vi "Create Actor.vi"(11 "QualifiedName":string="demo/producer") -> (0 "error out":errorcluster, 3 "Actor Class":T1)   [LabVIEW 2013]
uses:
  Actor Private Data.ctl
  <vilib>/LabVIEW Open Source Project/MQTT Client/Client class/Client.lvclass
  Actor Private Events -- cluster.ctl
  Payload -- cluster.ctl
  <vilib>/LabVIEW Open Source Project/OpenSerializer JKI JSON/Serializer.JSON.lvclass
  <vilib>/LabVIEW Open Source Project/MQTT Connection/MQTT_Base/Base Class/MQTT_Base.lvclass/MQTT_Base.ctl
  <vilib>/LabVIEW Open Source Project/MQTT Control Packets/Control Packets/PUBLISH/PUBLISH.lvclass
  <vilib>/LabVIEW Open Source Project/OpenSerializer/Serializer.FlattenedString/Serializer.FlattenedString.lvclass
  <vilib>/LabVIEW Open Source Project/OpenSerializer/Serializer/Serializer.lvclass
  <vilib>/LabVIEW Open Source Project/Connection/Connection.TCP/Connection.TCP.lvclass
  <vilib>/LabVIEW Open Source Project/MQTT Connection/MQTT_Base/Base Class/MQTT_Base.lvclass
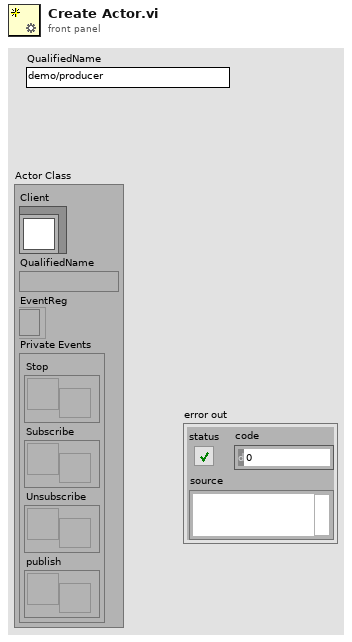
[diagram p1: front panel]
types:
  T1 = typedef "Actor Private Data.ctl" = cluster{"Client":refnum<class "Client.lvclass">, "QualifiedName":string, "EventReg":refnum<event-registration>, "Private Events":T2}
  T2 = typedef "Actor Private Events -- cluster.ctl" = cluster{"Stop":refnum<user-event>, "Subscribe":refnum<user-event>, "Unsubscribe":refnum<user-event>, "publish":refnum<user-event>}
  T3 = typedef "Payload -- cluster.ctl" = cluster{"topic":string, "Payload":u8[]}
  T4 = typedef "MQTT Base.lvlib/MQTT_Base.lvclass/Public Events -- cluster.ctl" = cluster{"Stop Event":refnum<user-event>, "Error Event":refnum<user-event>, "Inbound Message":refnum<user-event>}
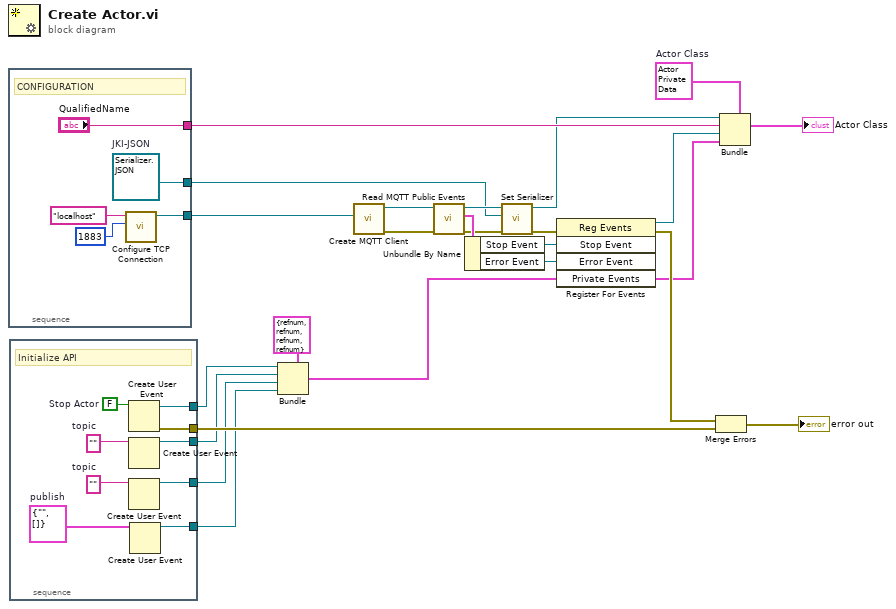
[diagram p0: block diagram]
diagram:
  w23 = T1 {"Client"=refnum, "QualifiedName"="", "EventReg"=refnum, "Private Events"={"Stop"=refnum, "Subscribe"=refnum, "Unsubscribe"=refnum, "publish"=refnum}}  # Actor Class
  n1 = stacked-sequence {
    tunnel: ["QualifiedName"] -> w22
    tunnel: [w26] -> w11
    tunnel: [w25] -> w10
    frame #0 {
      w25 = refnum<class "Serializer.JSON.lvclass"> refnum  # JKI-JSON
      # "CONFIGURATION"
      n2 = call <vilib>:"Configure TCP Connection.vi"("remote port (80)"=u16 1883, "address (localhost)"="localhost") -> ("Connection.TCP"=w26:refnum<class "Connection.TCP.lvclass">)  [unwired: 8 in, 1 out]
    }
  }
  n3 = stacked-sequence {
    tunnel: [w37] -> w20
    tunnel: [w36] -> w19
    tunnel: [w33] -> w3
    tunnel: [w32] -> w2
    tunnel: [w30] -> w1
    frame #0 {
      w31 = T3 {"topic"="", "Payload"=[]}  # publish
      w34 = ""  # topic
      w35 = ""  # topic
      w38 = FALSE  # Stop Actor
      # "Initialize API"
      n4 = Create User Event(user event datatype=w38) -> (user event=w37:refnum<user-event>, error out=w36:errorcluster)  [unwired: 1 in]
      n5 = Create User Event(user event datatype=w35) -> (user event=w33:refnum<user-event>)  [unwired: 1 in, 1 out]
      n6 = Create User Event(user event datatype=w34) -> (user event=w32:refnum<user-event>)  [unwired: 1 in, 1 out]
      n7 = Create User Event(user event datatype=w31) -> (user event=w30:refnum<user-event>)  [unwired: 1 in, 1 out]
    }
  }
  n8 = Bundle(cluster=T2 {"Stop"=refnum, "Subscribe"=refnum, "Unsubscribe"=refnum, "publish"=refnum} ("Private Events"), "Stop"=w20, "Subscribe"=w3, "Unsubscribe"=w2, "publish"=w1) -> (w7:T2)
  n9 = call <vilib>:"Create MQTT Client.vi"("Connection Configuration"=w11) -> ("error out"=w5:errorcluster, "Client out"=w6:refnum<class "Client.lvclass">)  [unwired: 9 in]
  n10 = call <vilib>:"Read MQTT Public Events.vi"("error in (no error)"=w5, "MQTT_Base in"=w6) -> ("error out"=w14:errorcluster, "MQTT Public Events"=w15:T4, "MQTT_Base out"=w12:refnum<class "Client.lvclass">)  [unwired: 7 in]
  n11 = Unbundle By Name(w15) -> ("Stop Event"=w17:refnum<user-event>, "Error Event"=w16:refnum<user-event>)
  n12 = call <vilib>:"Set Serializer.vi"("error in (no error)"=w14, "Serializer (default: Flattened String)"=w10, "MQTT_Base"=w12) -> ("error out"=w13:errorcluster, "MQTT_Base out"=w9:refnum<class "Client.lvclass">)  [unwired: 7 in]
  n13 = register-events(error in=w13, w17, w16, w7) -> (reference out=w4:refnum<event-registration>, error out=w8:errorcluster)  [unwired: 1 in]
  n14 = Merge Errors(w8, w19) -> (→"error out":errorcluster)
  n15 = Bundle(cluster=w23, "Client"=w9, "QualifiedName"=w22, "EventReg"=w4, "Private Events"=w7) -> (→"Actor Class":T1)
